vi "LuaVIEW Load Script File.vi"(0 "script file":path, 5 "custom search directory (none)":path, 11 "error in (no error)":errorcluster, 12 "loaded scripts in (none)":path[](array[path])) -> (4 "absolute path":path, 6 "have new script":bool, 8 "script text":string, 14 "loaded scripts out":path[](array[path]), 15 "error out":errorcluster)   [LabVIEW 2012]
doc: "Loads a script file given an absolute or relative path. In case of a relative path, any custom search directory, the directories of any loaded scripts, and any configured script directories (in that order) are prepended to construct absolute paths at which the script is attempted to be loaded. If none of these directories contains the specified script, an error is reported. The loaded script text has its end of line markers converted to linefeeds. In addition to providing a search path, the (optional) list of already loaded scripts also functions as an exclusion list so that the same script will not be loaded twice."
uses:
  glb_LuaVIEW Configuration Globals.vi
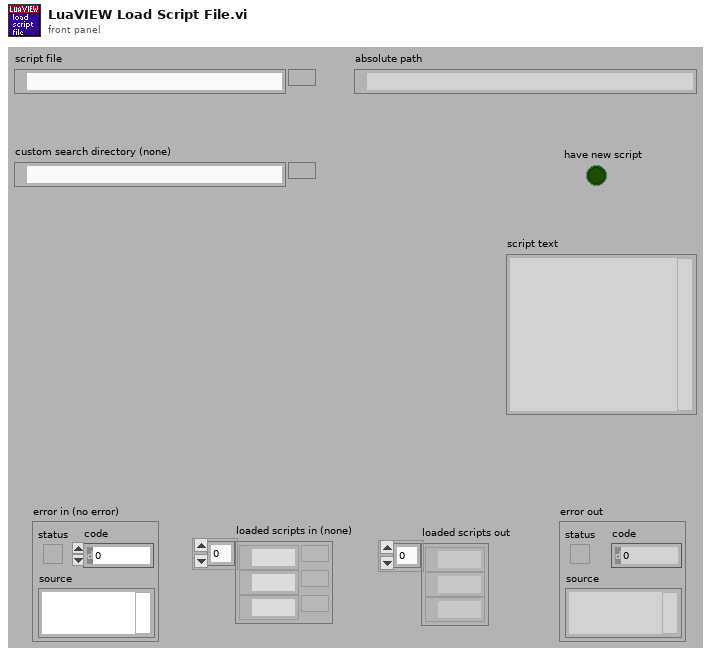
[diagram p1: front panel]
types:
  T1 = enum16{"read/write", "read-only", "write-only", "write-only (truncate)"}
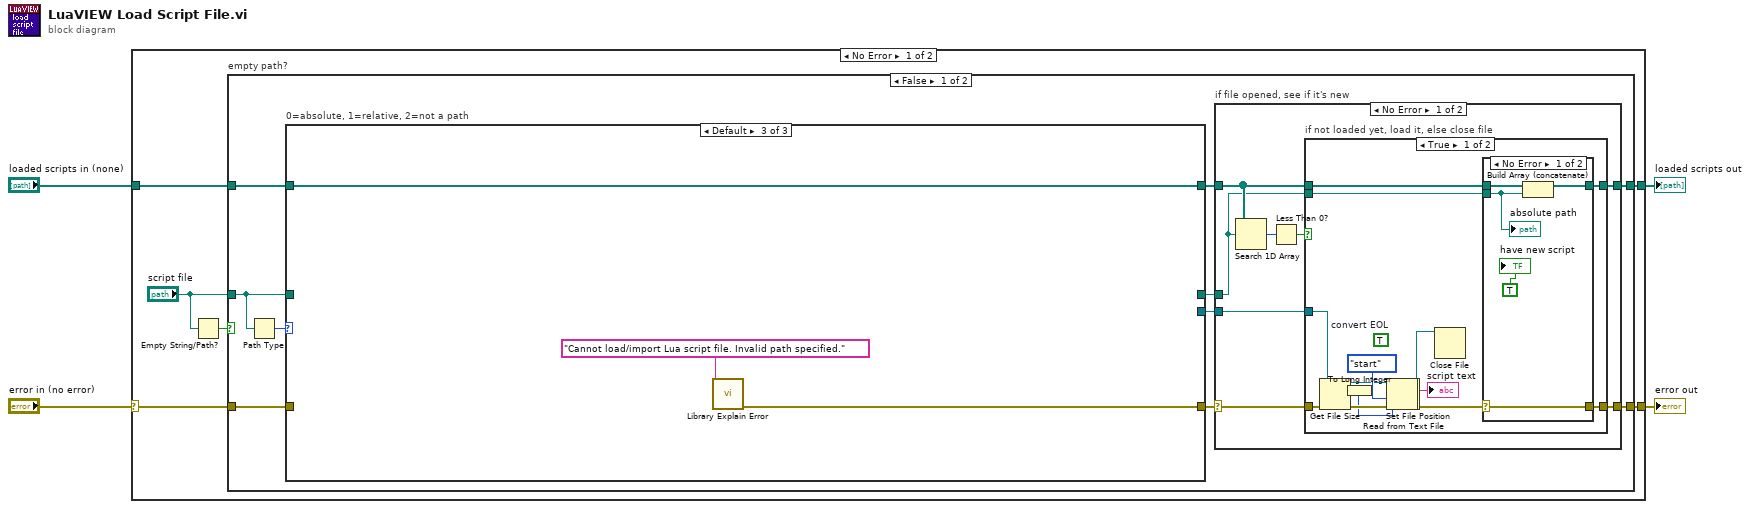
[diagram p0: block diagram]
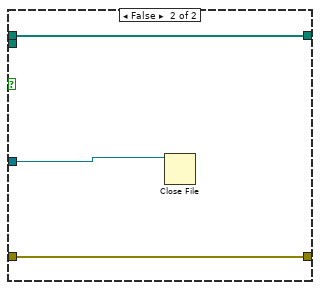
[diagram p3: hidden frame]
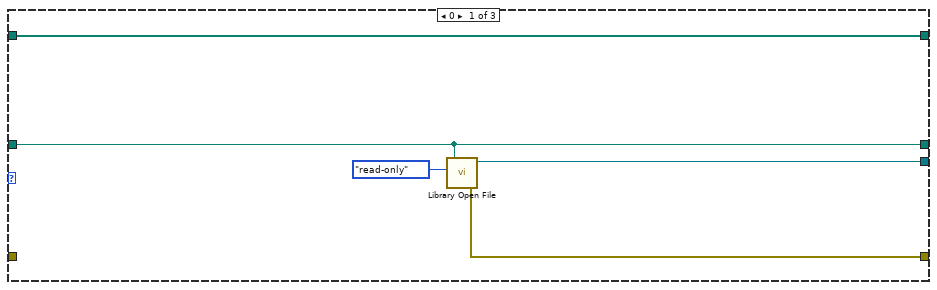
[diagram p5: hidden frame]
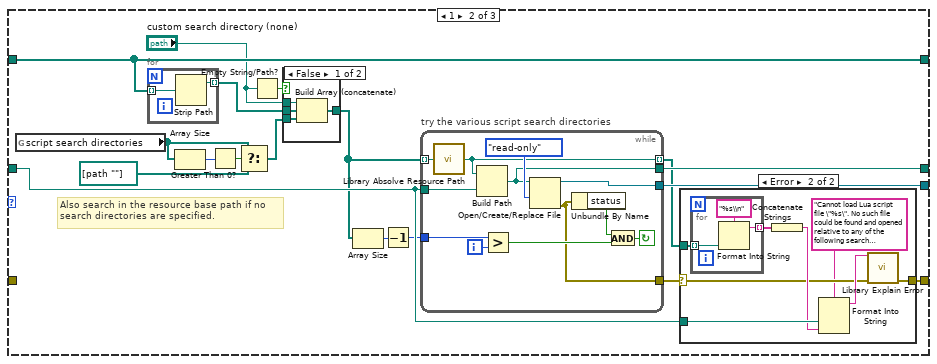
[diagram p6: hidden frame]
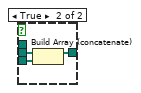
[diagram p8: hidden frame]
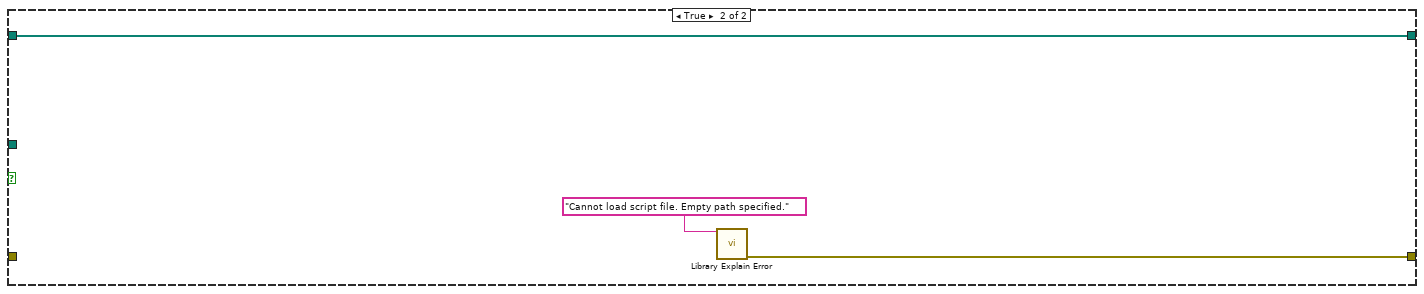
[diagram p9: hidden frame]
diagram:
  n1 = case shown="No Error" "error in (no error)" {
    selector: "error in (no error)" -> [w9 w120]
    tunnel: [w10 w120] -> w3
    tunnel: "loaded scripts in (none)" -> [w6 w119]
    tunnel: [w5 w119] -> w1
    frame No Error {
      n2 = Empty String/Path?(string/path="script file") -> (empty?=w8:bool)
      n3 = case "empty path?" shown="False" w8 {
        tunnel: "script file" -> [w19 _]
        tunnel: [w16 w118] -> w10
        tunnel: w9 -> [w18 _]
        tunnel: w6 -> [w12 w116]
        tunnel: [w14 w116] -> w5
        frame False {
          n4 = Path Type(1:w19) -> (0:w20:i16)
          n5 = case "0=absolute, 1=relative, 2=not a path" shown="Default" w20 {
            tunnel: [w61 w79 _] -> w13
            tunnel: w19 -> [w61 w76 _]
            tunnel: [w59 w77 w114] -> w17
            tunnel: w18 -> [_ _ _]
            tunnel: [w60 w78 _] -> w15
            tunnel: w12 -> [w57 w75 w113]
            tunnel: [w57 w75 w113] -> w11
            frame 0 {
              n6 = call "Library Open File.vi"("open mode (read/write)"=T1."read-only", "file path"=w61) -> ("error out"=w59:errorcluster, "refnum"=w60:refnum<file>)  [unwired: 4 in]
            }
            frame 1 {
              # "Also search in the resource base path if no\nsearch directories are specified."
              n7 = global read "glb_LuaVIEW Configuration Globals.vi" "script search directories"() -> (w66:path[])
              n8 = for {
                tunnel: w75 -> [w112] mode=indexing
                tunnel: [w111] -> w74 mode=indexing
                n9 = Strip Path(path=w112) -> (stripped path=w111:path)  [unwired: 1 out]
              }
              n10 = Array Size(array=w66) -> (size(s)=w69:i32)
              n11 = Greater Than 0?(x=w69) -> (x > 0?=w68:bool)
              n12 = Select(t=w66, s=w68, f=path[] [path ""] ("array")) -> (s? t:f=w65:path[])
              n13 = Empty String/Path?(string/path="custom search directory (none)") -> (empty?=w72:bool)
              n14 = case shown="False" w72 {
                tunnel: w65 -> [w107 w110]
                tunnel: w74 -> [w106 w109]
                tunnel: [w104 w108] -> w73
                tunnel: "custom search directory (none)" -> [w105 _]
                frame False {
                  n15 = Build Array (concatenate)(w105, w106, w107) -> (w104:path[])
                }
                frame True {
                  n16 = Build Array (concatenate)(w109, w110) -> (w108:path[])
                }
              }
              n17 = Array Size(array=w73) -> (size(s)=w70:i32)
              n18 = Decrement(x=w70) -> (x-1=w64:i32)
              n19 = while "try the various script search directories" {
                tunnel: w73 -> [w94] mode=indexing
                tunnel: w64 -> [w103]
                tunnel: [w100] -> w78
                tunnel: w76 -> [w99]
                tunnel: [w98] -> w79
                tunnel: [w93] -> w63 mode=indexing
                tunnel: [w92] -> w62
                i -> [w102]
                stop <- w96 continue-if-true
                n20 = call "Library Absolve Resource Path.vi"("path in"=w94) -> ("absolved path"=w93:path)  [unwired: 14 in]
                n21 = Build Path(base path=w93, name or relative path=w99) -> (appended path=w98:path)
                n22 = Greater?(x=w103, y=w102) -> (0:w97:bool)
                n23 = Open/Create/Replace File(file path (use dialog)=w98, access (0:read/write)=T1."read-only" ("open mode (0)")) -> (refnum out=w100:refnum<file>, error out=w92:errorcluster)  [unwired: 4 in, 1 out]
                n24 = Unbundle By Name(w92) -> ("status"=w95:bool)
                n25 = And(x=w95, y=w97) -> (x .and. y?=w96:bool)
              }
              n26 = case shown="Error" w62 {
                selector: w62 -> [w80 w82]
                tunnel: w76 -> [_ w87]
                tunnel: [w80 w86] -> w77
                tunnel: w63 -> [_ w85]
                frame No Error {
                }
                frame Error {
                  n27 = for {
                    tunnel: w85 -> [w91] mode=indexing
                    tunnel: [w89] -> w84 mode=indexing
                    n28 = Format Into String(format string="%s\\n", w91) -> (resulting string=w89:string)  [unwired: 2 in, 1 out]
                  }
                  n29 = Concatenate Strings(w84) -> (w83:string)
                  n30 = Format Into String(format string="Cannot load Lua script file \"%s\". No such file could be found and opened relative to any of the following search directories:\n%s", w87, w83) -> (resulting string=w88:string)  [unwired: 2 in, 1 out]
                  n31 = call "Library Explain Error.vi"("explanation prefix (none)"=w88, "error in (no error)"=w82) -> ("explained error"=w86:errorcluster)  [unwired: 13 in]
                }
              }
            }
            frame Default {
              n32 = call "Library Explain Error.vi"("explanation prefix (none)"="Cannot load/import Lua script file. Invalid path specified." ("explanation")) -> ("explained error"=w114:errorcluster)  [unwired: 14 in]
            }
          }
          n33 = case "if file opened, see if it's new" shown="No Error" w17 {
            selector: w17 -> [w26 w56]
            tunnel: [w27 w56] -> w16
            tunnel: w15 -> [w28 _]
            tunnel: w11 -> [w23 w55]
            tunnel: [w21 w55] -> w14
            tunnel: w13 -> [w22 _]
            frame No Error {
              n34 = Search 1D Array(1D array=w23, element=w22) -> (index of element=w25:i32)  [unwired: 1 in]
              n35 = Less Than 0?(x=w25) -> (x < 0?=w24:bool)
              n36 = case "if not loaded yet, load it, else close file" shown="True" w24 {
                tunnel: w28 -> [w43 w54]
                tunnel: [w37 w53] -> w27
                tunnel: w26 -> [w32 w53]
                tunnel: w23 -> [w35 w52]
                tunnel: w22 -> [w33 _]
                tunnel: [w34 w52] -> w21
                frame True {
                  (unwired) TRUE  # convert EOL
                  n37 = Get File Size(file=w43, error in=w32) -> (refnum out=w42:refnum<file>, size (in bytes)=w31:i64, 0:w41:errorcluster)
                  n38 = To Long Integer(number=w31) -> (32bit integer=w40:i32)
                  n39 = Set File Position(refnum=w42, from (0:start)=enum16{"start", "end", "current"}."start" ("pos mode (0:2)"), error in=w41) -> (refnum out=w30:refnum<file>, error out=w29:errorcluster)  [unwired: 1 in]
                  n40 = Read from Text File(file (use dialog)=w30, count=w40, error in=w29) -> (refnum out=w39:refnum<file>, text=→"script text":string, error out=w36:errorcluster)  [unwired: 1 in, 1 out]
                  n41 = Close File(refnum=w39) -> ()  [unwired: 1 in, 2 out]
                  n42 = case shown="No Error" w36 {
                    selector: w36 -> [w49 w51]
                    tunnel: [w49 w51] -> w37
                    tunnel: w35 -> [w48 w50]
                    tunnel: [w47 w50] -> w34
                    tunnel: w33 -> [w46 _]
                    frame No Error {
                      n43 = Build Array (concatenate)(w48, w46) -> (w47:path[])
                      "have new script" <- TRUE
                      "absolute path" <- w46
                    }
                    frame Error {
                    }
                  }
                }
                frame False {
                  n44 = Close File(refnum=w54) -> ()  [unwired: 1 in, 2 out]
                }
              }
            }
            frame Error {
            }
          }
        }
        frame True {
          n45 = call "Library Explain Error.vi"("explanation prefix (none)"="Cannot load script file. Empty path specified." ("explanation")) -> ("explained error"=w118:errorcluster)  [unwired: 14 in]
        }
      }
    }
    frame Error {
    }
  }
  "error out" <- w3
  "loaded scripts out" <- w1
